vi "createConfig.vi"(8 "error in (no error)":errorcluster, 11 "SMO in":refnum<class "SMO.lvclass">) -> (0 "error out":errorcluster, 3 "SMO out":refnum<class "SMO.lvclass">)   [LabVIEW 2019, in "SMO.lvclass"]
doc: "JKI State Machine Objects (SMO) 1.3.0.56\nJKI - JKI\nCopyright (c) 2017, JKI"
uses:
  SMO.lvclass
  Support/Attribute.Config/Attribute.Config.lvclass/Attribute.Config.ctl
  Support/Attribute.Config/AccessScope.ctl
  SMO.lvclass/SMO.ctl
  Support/Attribute.Config/Attribute.Config.lvclass
  C:/Users/Patrick/Documents/GitHub/Test (LV2019)/lv-venv/lv.lib/vi.lib/JKI/JKI SMO/Support/Attribute/Attribute.lvclass
  Support/Attribute/Attribute.lvclass
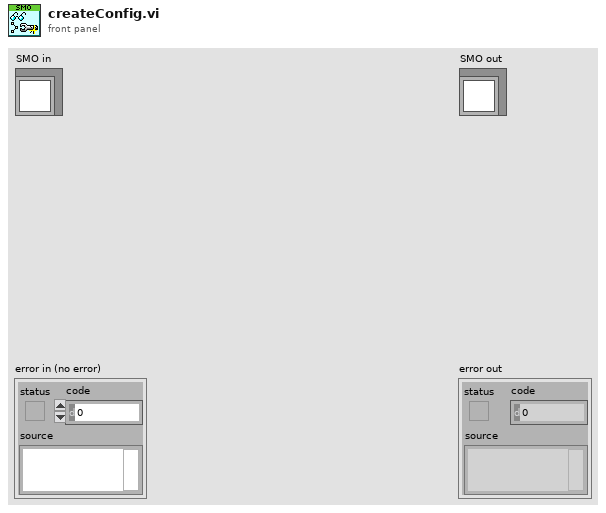
[diagram p1: front panel]
types:
  T1 = typedef "Attribute.Config.lvclass/AccessScope.ctl" = enum16{"RO", "RW"}
  T2 = typedef "SMO.lvclass/PrivateData--Ref.ctl" = refnum<data-value>
  T3 = typedef "SMO.lvclass/PrivateData--Cluster.ctl" = cluster{"Parent Call":T4, "Registered Processes":T5[], "Sync Notifier":refnum<notifier>, "Process Error Notifier":refnum<notifier>, "Protected Events":T6, "Public Events":T7, "SMO State":T8, "[Dependencies]":T9[], "[Attributes]":refnum<class "Attribute.lvclass">[], "Launcher Close":refnum<notifier>, "Caller Watchdog":refnum<queue>, "Accessibility":T10, "NbStaticDependencies":u32}
  T4 = typedef "SMO.lvclass/Parent Call--Enum.ctl" = enum16{"Allows parent to run", "Does not request parent to run"}
  T5 = typedef "SMO.lvclass/RegisteredProcessData--Cluster.ctl" = cluster{"Name":string, "Static VI Ref":refnum<vi>, "Running":bool, "NotifierRef":u32}
  T6 = typedef "SMO.lvclass/Protected Events.ctl" = cluster{"StopProcesses":refnum<user-event>, "AbortProcesses":refnum<user-event>, "Config Changed":refnum<user-event>, "Dependency":refnum<user-event>}
  T7 = typedef "SMO.lvclass/Public Events.ctl" = cluster{"Error":refnum<user-event>, "State":refnum<user-event>, "Reserve State":refnum<user-event>}
  T8 = typedef "SMO.lvclass/SMOState --Enum.ctl" = enum16{"unknown", "Created", "Started", "Stopped"}
  T9 = typedef "SMO.lvclass/SMO Dependency--Cluster.ctl" = cluster{"Dependency":refnum<class "SMO.lvclass">, "Level":string}
  T10 = typedef "SMO.lvclass/Accessibility--Cluster.ctl" = cluster{"Lock Key":string, "Reserve State":T11}
  T11 = typedef "SMO.lvclass/Reserve State--Enum.ctl" = enum16{"Unreserved", "Reserved", "Self-locked"}
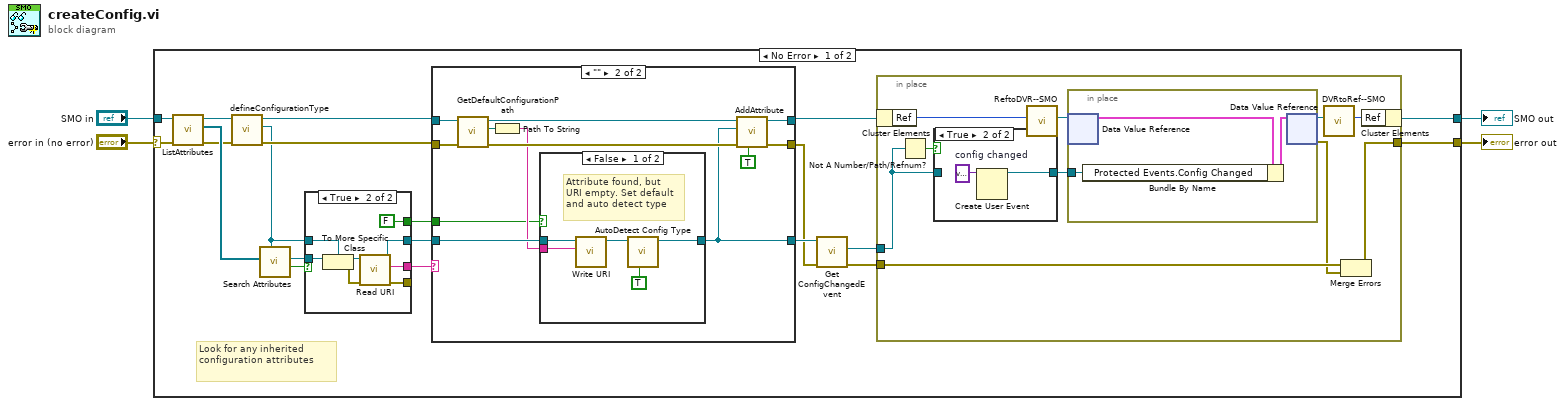
[diagram p0: block diagram]
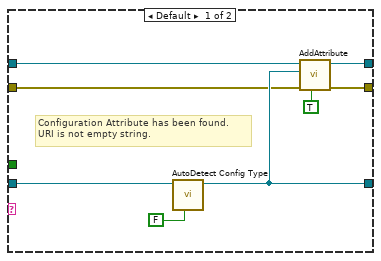
[diagram p3: hidden frame]
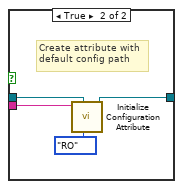
[diagram p4: hidden frame]
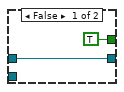
[diagram p5: hidden frame]
diagram:
  n1 = case shown="No Error" "error in (no error)" {
    selector: "error in (no error)" -> [w21 w81]
    tunnel: [w11 w81] -> w3
    tunnel: [w15 w80] -> w1
    tunnel: "SMO in" -> [w23 w80]
    frame No Error {
      # "Look for any inherited configuration attributes"
      n2 = call "ListAttributes.vi"("error in (no error)"=w21, "SMO in"=w23) -> ("error out"=w7:errorcluster, "[Attributes]"=w22:refnum<class "Attribute.lvclass">[], "SMO out"=w9:refnum<class "SMO.lvclass">)  [unwired: 7 in]
      n3 = call-dynamic "defineConfigurationType.vi"("error in (no error)"=w7, "SMO in"=w9) -> ("error out"=w6:errorcluster, "Attribute.Config"=w5:refnum<class "Attribute.Config.lvclass">, "SMO out"=w8:refnum<class "SMO.lvclass">)  [unwired: 7 in]
      n4 = call "Search Attributes.vi"("Attribute type"=w5, "[Attributes]"=w22) -> ("found"=w20:bool, "Attribute out"=w24:refnum<class "Attribute.lvclass">)  [unwired: 8 in]
      n5 = case shown="True" w20 {
        tunnel: w24 -> [_ w79]
        tunnel: w5 -> [w71 w78]
        tunnel: [_ w75] -> w19
        tunnel: [_ w74] -> _
        tunnel: [w71 w73] -> w18
        tunnel: [TRUE FALSE] -> w17
        frame False {
        }
        frame True {
          n6 = To More Specific Class(target class=w78, reference=w79) -> (specific class reference=w77:refnum<class "Attribute.Config.lvclass">, error out=w76:errorcluster)  [unwired: 1 in]
          n7 = call "Read URI.vi"("error in (no error)"=w76, "Attribute.Config in"=w77) -> ("error out"=w74:errorcluster, "URI"=w75:string, "Attribute.Config out"=w73:refnum<class "Attribute.Config.lvclass">)  [unwired: 7 in]
        }
      }
      n8 = case shown="\"\"" w19 {
        tunnel: w8 -> [w44 w60]
        tunnel: [w43 w55] -> w14
        tunnel: w6 -> [w42 w59]
        tunnel: [w41 w53] -> w13
        tunnel: w18 -> [w48 w58]
        tunnel: w17 -> [_ w49]
        tunnel: [w45 w52] -> w16
        frame Default {
          # "Configuration Attribute has been found.\nURI is not empty string."
          n9 = call-dynamic "AutoDetect Config Type.vi"("overwrite type (F)"=FALSE, "Attribute.Config in"=w48) -> ("Attribute.Config out"=w45:refnum<class "Attribute.Config.lvclass">)  [unwired: 8 in, 1 out]
          n10 = call "AddAttribute.vi"("Overwrite? (F)"=TRUE, "error in (no error)"=w42, "Attribute"=w45, "SMO in"=w44) -> ("error out"=w41:errorcluster, "SMO out"=w43:refnum<class "SMO.lvclass">)  [unwired: 6 in]
        }
        frame "" {
          n11 = call-dynamic "GetDefaultConfigurationPath.vi"("error in (no error)"=w59, "SMO in"=w60) -> ("error out"=w54:errorcluster, "Default Configuration Path"=w57:path, "SMO out"=w56:refnum<class "SMO.lvclass">)  [unwired: 7 in]
          n12 = Path To String(path=w57) -> (string=w51:string)
          n13 = case shown="False" w49 {
            tunnel: w58 -> [w65 w69]
            tunnel: [w62 w68] -> w52
            tunnel: w51 -> [w64 w66]
            frame False {
              # "Attribute found, but\nURI empty. Set default\nand auto detect type"
              n14 = call "Write URI.vi"("URI"=w64, "Attribute.Config in"=w65) -> ("Attribute.Config out"=w63:refnum<class "Attribute.Config.lvclass">)  [unwired: 8 in, 1 out]
              n15 = call-dynamic "AutoDetect Config Type.vi"("overwrite type (F)"=TRUE, "Attribute.Config in"=w63) -> ("Attribute.Config out"=w62:refnum<class "Attribute.Config.lvclass">)  [unwired: 8 in, 1 out]
            }
            frame True {
              # "Create attribute with\ndefault config path"
              n16 = call "Initialize Configuration Attribute.vi"("Access Scope (RO)"=AccessScope."RO", "Attribute.Config in"=w69, "URI"=w66) -> ("Attribute.Config"=w68:refnum<class "Attribute.Config.lvclass">)  [unwired: 7 in, 1 out]
            }
          }
          n17 = call "AddAttribute.vi"("Overwrite? (F)"=TRUE, "error in (no error)"=w54, "Attribute"=w52, "SMO in"=w56) -> ("error out"=w53:errorcluster, "SMO out"=w55:refnum<class "SMO.lvclass">)  [unwired: 6 in]
        }
      }
      n18 = call "Get ConfigChangedEvent.vi"("error in (no error)"=w13, "Attribute.Config in"=w16) -> ("error out"=w12:errorcluster, "Config change event"=w10:refnum<user-event>)  [unwired: 7 in, 1 out]
      n19 = in-place {
        in-place-border: w12 -> [w30]
        in-place-border: [w28] -> w11
        in-place-border: w10 -> [w25]
        n20 = in-place-cluster #1(w14) -> ("Ref"=w34:u32)
        n21 = Not A Number/Path/Refnum?(number/path/refnum=w25) -> (NaN/Path/Refnum?=w27:bool)
        n22 = case shown="True" w27 {
          tunnel: [w35 w36] -> w26
          tunnel: w25 -> [w35 _]
          frame False {
          }
          frame True {
            w37 = variant  # config changed
            n23 = Create User Event(user event datatype=w37) -> (user event=w36:refnum<user-event>)  [unwired: 1 in, 1 out]
          }
        }
        n24 = call "ReftoDVR--SMO.vi"("Ref"=w34) -> ("Ref"=w33:T2)  [unwired: 10 in]
        n25 = in-place {
          in-place-border: w26 -> [w38]
          n26 = in-place-dvr #2(w33) -> (w40:T3)  [unwired: 1 out]
          n27 = Bundle By Name(cluster=w40, "Protected Events.Config Changed"=w38) -> (w39:T3)
          n28 = in-place-dvr #2(w39) -> (w32:T2, w29:errorcluster)
        }
        n29 = call "DVRtoRef--SMO.vi"("Ref"=w32) -> ("Ref"=w31:u32)  [unwired: 10 in]
        n30 = Merge Errors(w30, w29) -> (w28:errorcluster)
        n31 = in-place-cluster #1("Ref"=w31) -> (w15:refnum<class "SMO.lvclass">)
      }
    }
    frame Error {
    }
  }
  "error out" <- w3
  "SMO out" <- w1
